vi "UDP Multicast Write-Only Open.vi"(7 "net address":u32, 8 "error in (no error)":errorcluster, 9 "time-to-live (1)":u16=1, 11 "port":u16) -> (0 "error out":errorcluster, 3 "connection ID":refnum<k16>)   [LabVIEW 2018]
doc: "Opens a UDP multicast socket on the <B>port</B>. You must manually select the polymorphic instance you want to use."
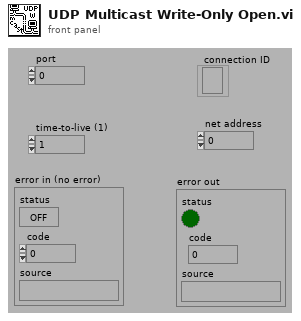
[diagram p1: front panel]
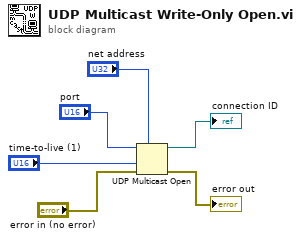
[diagram p0: block diagram]
diagram:
  n1 = UDP Multicast Open(7:"net address", 8:"error in (no error)", 9:"time-to-live (1)", 11:"port") -> (0:→"error out":errorcluster, 3:→"connection ID":refnum<k16>)  [unwired: 2 out]
